vi "image display.vi"(0 "webcam":T1) -> (14 "red out":u32[](array[numeric]), 15 "green out":u32[](array[numeric]), 16 "blue out":u32[](array[numeric]), 17 "original":T2(plugin-control), 18 "X Resolution":i32, 19 "Y Resolution":i32)   [LabVIEW 2019]
uses:
  <vilib>/userDefined/High Color/IMAQdx.ctl
  <vilib>/vision/NI_Vision_Development_Module.lvlib
  <vilib>/vision/driver/NI_Vision_Acquisition_Software.lvlib
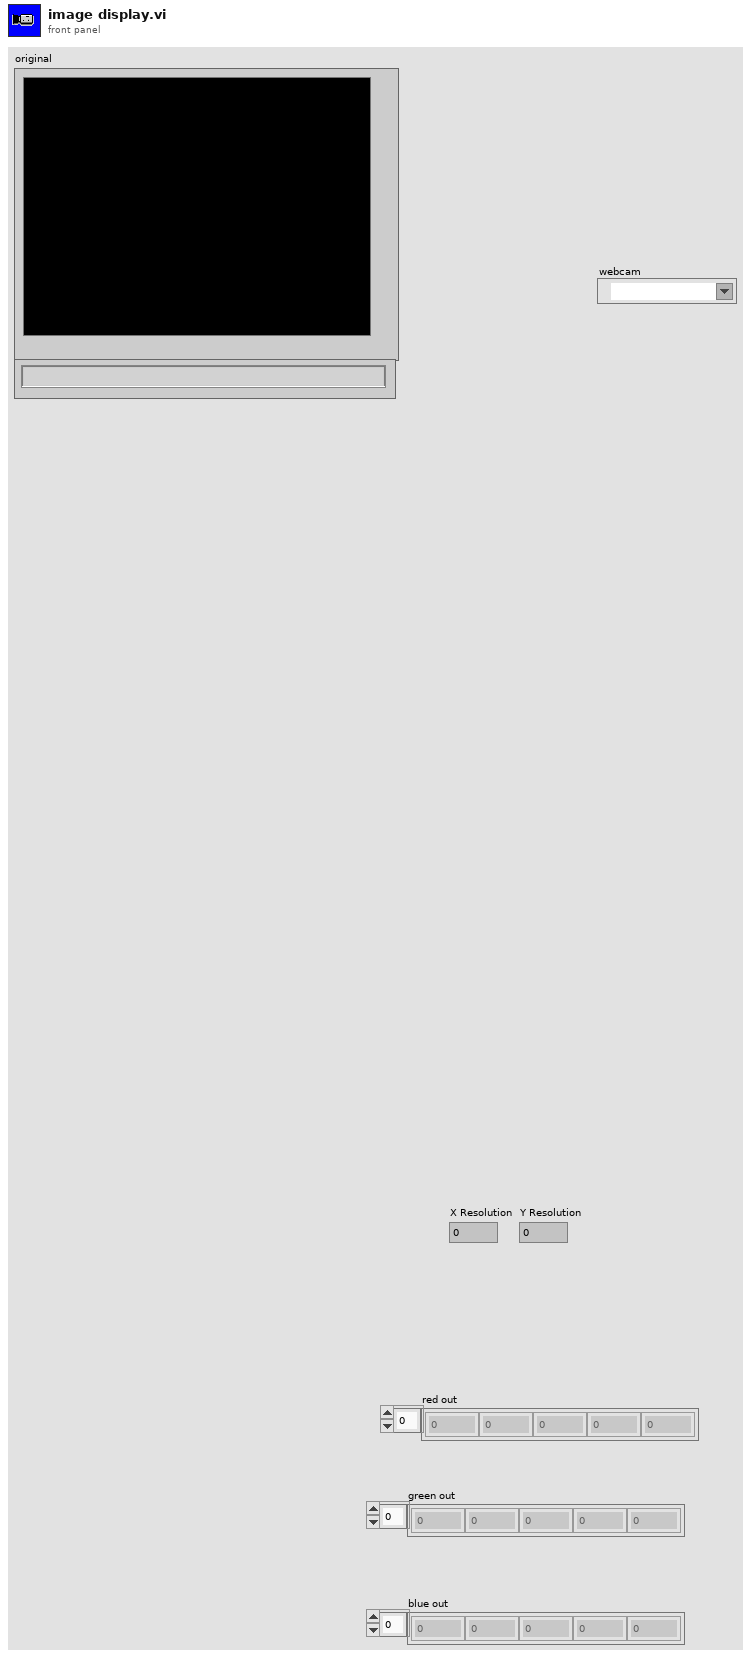
[diagram p1: front panel]
types:
  T1 = typedef "IMAQdx.ctl" = refnum<k21>
  T2 = typedef "IMAQ Image.ctl" = refnum<image>
  T3 = typedef "Image Type" = u32
  T4 = cluster{"Red (or Hue) value":u8, "Green (or Sat) value":u8, "Blue (or Light or Val) value":u8}
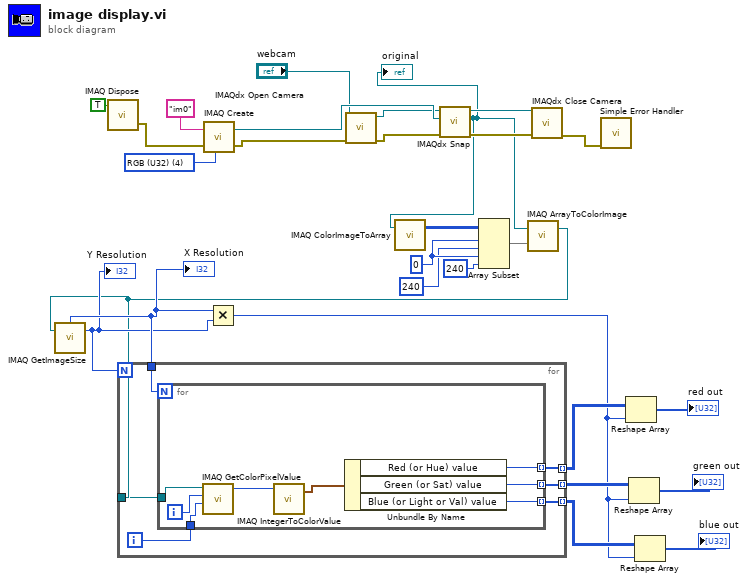
[diagram p0: block diagram]
diagram:
  w8 = T3 4 items=["Grayscale (U8)", "Grayscale (I16)", "Grayscale (SGL)", "Complex (CSG)", "RGB (U32)", "HSL (U32)", "RGB (U64)", "Grayscale (U16)"] ("Image Type")
  w14 = 0
  n1 = call "IMAQ Dispose"("All Images? (No)"=TRUE) -> ("error out"=w3:errorcluster)  [unwired: 5 in]
  n2 = call "IMAQ Create"("Image Name"="im0", "Image Type"=w8, "error in (no error)"=w3) -> ("New Image"=w18:T2, "error out"=w19:errorcluster)  [unwired: 1 in, 1 out]
  n3 = call <vilib>:"IMAQdx Open Camera.vi"("error in"=w19, "Session In"="webcam") -> ("error out"=w5:errorcluster, "Session Out"=w6:T1)  [unwired: 8 in]
  n4 = call <vilib>:"IMAQdx Snap.vi"("error in"=w5, "Image In"=w18, "Session In"=w6) -> ("error out"=w15:errorcluster, "Image Out"=w9:T2, "Session Out"=w16:T1)  [unwired: 6 out]
  "original" <- w9
  n5 = call "IMAQ ColorImageToArray"("Image"=w9) -> ("Image Pixels (U32)"=w12:u32[][])  [unwired: 3 in, 2 out]
  n6 = Array Subset(array=w12, index (row)=w14, length (row)=240 ("length"), index (col)=w14, length (col)=240) -> (w11:u32[][])
  n7 = call "IMAQ ArrayToColorImage"("Image Pixels (U32)"=w11, "Image"=w9) -> ("Image Out"=w1:T2)  [unwired: 3 in, 1 out]
  n8 = call "IMAQ GetImageSize"("Image"=w1) -> ("Y Resolution"=w22:i32, "X Resolution"=w23:i32)  [unwired: 3 in, 1 out]
  "X Resolution" <- w23
  "Y Resolution" <- w22
  n9 = for {
    N: w22 -> [_]
    tunnel: w1 -> [w34]
    tunnel: [w32] -> w27 mode=indexing
    tunnel: [w31] -> w25 mode=indexing
    tunnel: [w30] -> w26 mode=indexing
    tunnel: w23 -> [w29]
    i -> [w33]
    n10 = for {
      N: w29 -> [_]
      tunnel: w34 -> [w42]
      tunnel: w33 -> [w39]
      tunnel: [w38] -> w32 mode=indexing
      tunnel: [w37] -> w31 mode=indexing
      tunnel: [w36] -> w30 mode=indexing
      i -> [w35]
      n11 = call "IMAQ GetColorPixelValue"("Y Coordinate"=w39, "X Coordinate"=w35, "Image"=w42) -> ("Pixel Value (U32)"=w40:u32)  [unwired: 1 in, 2 out]
      n12 = call "IMAQ IntegerToColorValue"("U32 value"=w40) -> ("Color Value"=w41:T4)  [unwired: 4 in, 3 out]
      n13 = Unbundle By Name(w41) -> ("Red (or Hue) value"=w38:u8, "Green (or Sat) value"=w37:u8, "Blue (or Light or Val) value"=w36:u8)
    }
  }
  n14 = Multiply(x=w23, y=w22) -> (x*y=w24:i32)
  n15 = call <vilib>:"IMAQdx Close Camera.vi"("error in"=w15, "Session In"=w16) -> ("error out"=w17:errorcluster)  [unwired: 9 in]
  n16 = call <vilib>:"Simple Error Handler.vi"("error in (no error)"=w17) -> ()  [unwired: 4 in, 5 out]
  n17 = Reshape Array(w27, w24) -> (→"red out":u8[])
  n18 = Reshape Array(w25, w24) -> (→"green out":u8[])
  n19 = Reshape Array(w26, w24) -> (→"blue out":u8[])
